vi "ReadCAlexFile.vi"(7 "ExtraWeight(kg)":cluster{"Thigh":dbl, "Shank":dbl}, 8 "error in (no error)":errorcluster, 10 "ExpData File Path":path, 11 "CAlexData2":refnum<class "CAlex2_Data.lvclass">) -> (0 "error out":errorcluster, 3 "CAlexData 2":refnum<class "CAlex2_Data.lvclass">, 5 "CAlexVersion":T1)   [LabVIEW 2016, in "CAlex2_Data.lvclass"]
uses:
  CAlex2_Data.lvclass
  E:/LabVIEW.git/CAlex2-controller-master/Sim&Process/DataProcess/ExpData/ExpData.lvclass
  Classes/CAlex2/TypeDef/CAlexVersion.ctl
  Classes/CAlex2/CAlex2.lvclass
  Classes/CAlex2/TypeDef/LowerBodyDim.ctl
  CAlex2_Data.lvclass/CAlex2_Data.ctl
  ExpData/ExpData.lvclass
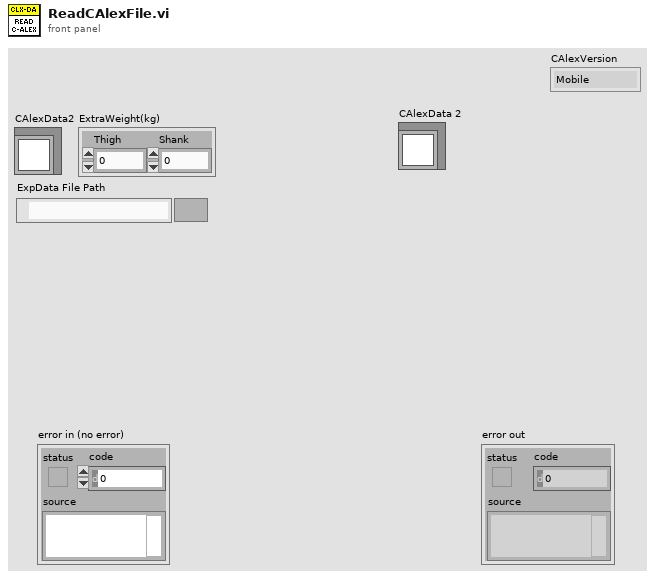
[diagram p1: front panel]
types:
  T1 = typedef "CAlex2.lvclass/CAlexVersion.ctl" = enum16{"Mobile", "Treadmill"}
  T2 = typedef "CAlex2.lvclass/LowerBodyDim.ctl" = cluster{"BodyDim":cluster{"ThighLt (m)":dbl, "ShankLt (m)":dbl, "HipWd (m)":dbl}, "BodyWt":cluster{"Thigh (kg)":dbl, "Shank (kg)":dbl}, "Cuff Loc":cluster{"HipCuffWd (m)":dbl, "HipCuffHt (m)":dbl, "HipFwdShift (m)":dbl, "ThighToKnee (m)":dbl, "ThighCuffDist (m)":dbl, "ShankToKnee (m)":dbl}}
  T3 = cluster{"[0]":dbl, "[1]":dbl, "[2]":dbl, "[3]":dbl, "[4]":dbl, "[5]":dbl}
  T4 = cluster{"array type (2D Dbl)[0]":dbl, "array type (2D Dbl)[1]":dbl, "array type (2D Dbl)[2]":dbl, "array type (2D Dbl)[3]":dbl, "array type (2D Dbl)[4]":dbl, "array type (2D Dbl)[5]":dbl}
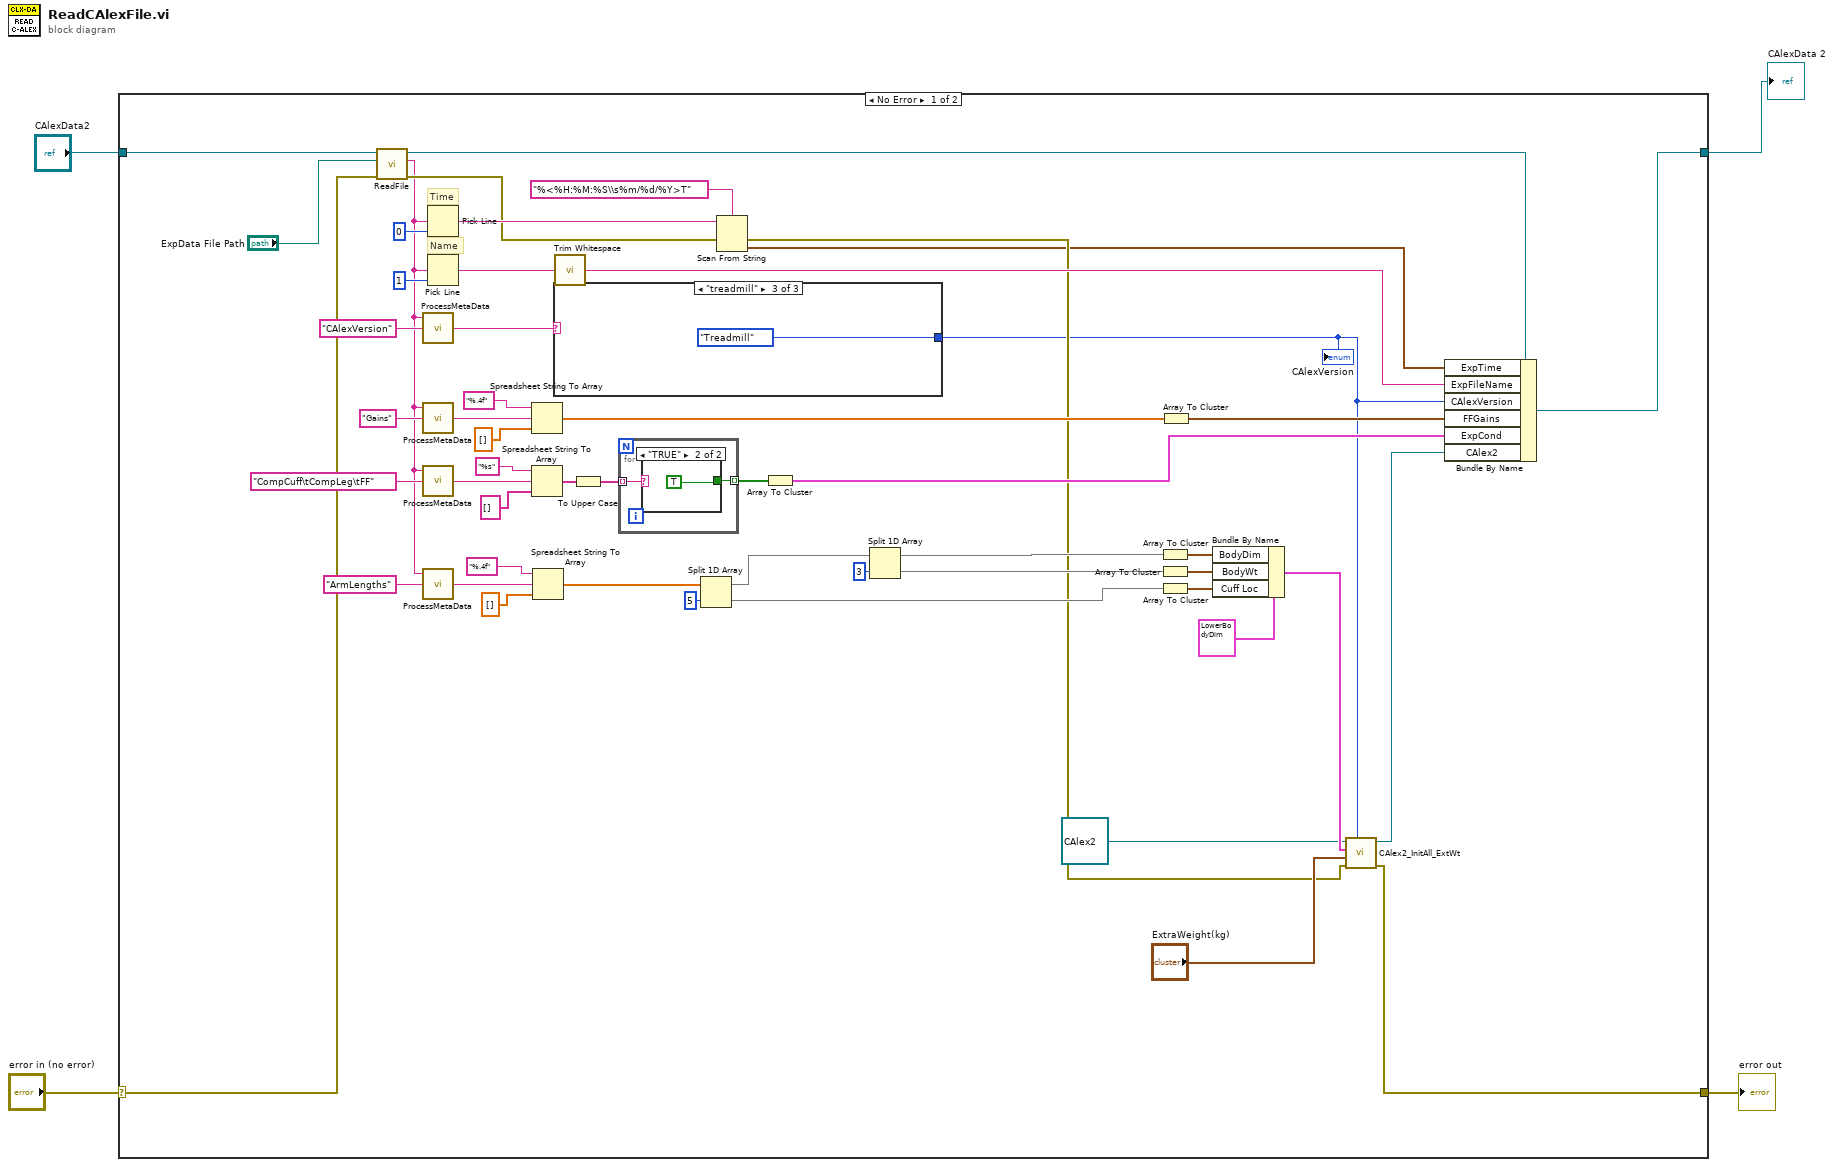
[diagram p0: block diagram]
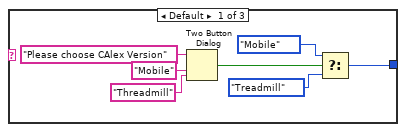
[diagram p2: hidden frame]
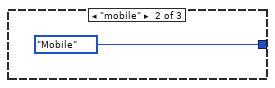
[diagram p3: hidden frame]
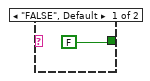
[diagram p4: hidden frame]
diagram:
  n1 = case shown="No Error" "error in (no error)" {
    selector: "error in (no error)" -> [w44 w71]
    tunnel: [w26 w71] -> w3
    tunnel: [w23 w70] -> w1
    tunnel: "CAlexData2" -> [w25 w70]
    frame No Error {
      # "Name"
      # "Time"
      n2 = call "ReadFile.vi"("error in (no error)"=w44, "ExpData File Path"="ExpData File Path", "ExpData In"=w25) -> ("error out"=w45:errorcluster, "MetaData"=w10:string, "ExpData Out"=w24:refnum<class "CAlex2_Data.lvclass">)  [unwired: 5 in, 1 out]
      n3 = call "ProcessMetaData.vi"("Header"="CAlexVersion", "MetaData"=w10) -> ("Data"=w6:string)  [unwired: 1 in]
      n4 = call "ProcessMetaData.vi"("Header"="Gains", "MetaData"=w10) -> ("Data"=w15:string)  [unwired: 1 in]
      n5 = call "ProcessMetaData.vi"("Header"="CompCuff\tCompLeg\tFF", "MetaData"=w10) -> ("Data"=w13:string)  [unwired: 1 in]
      n6 = call "ProcessMetaData.vi"("Header"="ArmLengths", "MetaData"=w10) -> ("Data"=w16:string)  [unwired: 1 in]
      n7 = Pick Line(multi-line string=w10, line index=0) -> (output string=w52:string)  [unwired: 1 in]
      n8 = Pick Line(multi-line string=w10, line index=1) -> (output string=w53:string)  [unwired: 1 in]
      n9 = Spreadsheet String To Array(format string="%.4f" ("format (%.3f)"), spreadsheet string=w15, array type (2D Dbl)=dbl[] []) -> (array=w43:dbl[])  [unwired: 1 in]
      n10 = Spreadsheet String To Array(format string="%s", spreadsheet string=w13, array type (2D Dbl)=string[] []) -> (array=w19:string[])  [unwired: 1 in]
      n11 = Spreadsheet String To Array(format string="%.4f" ("format (%.3f)"), spreadsheet string=w16, array type (2D Dbl)=dbl[] []) -> (array=w48:dbl[])  [unwired: 1 in]
      n12 = case shown="\"treadmill\"" w6 {
        tunnel: [w57 CAlexVersion."Mobile" ("CAlexVersion") CAlexVersion."Treadmill" ("CAlexVersion")] -> w5
        frame Default {
          n13 = Two Button Dialog(message="Please choose CAlex Version", 1:"Threadmill" ("F button name (\"Cancel\")"), 2:"Mobile" ("T button name (\"OK\")")) -> (T button?=w60:bool)
          n14 = Select(t=CAlexVersion."Mobile" ("CAlexVersion"), s=w60, f=CAlexVersion."Treadmill" ("CAlexVersion")) -> (s? t:f=w57:T1)
        }
        frame "mobile" {
        }
        frame "treadmill" {
        }
      }
      "CAlexVersion" <- w5
      n15 = call <vilib>:"Trim Whitespace.vi"("string"=w53) -> ("trimmed string"=w50:string)  [unwired: 1 in]
      n16 = To Upper Case(1:w19) -> (0:w18:string[])
      n17 = for {
        tunnel: w18 -> [w67] mode=indexing
        tunnel: [w66] -> w35 mode=indexing
        n18 = case shown="\"TRUE\"" w67 {
          tunnel: [FALSE TRUE] -> w66
          frame "FALSE", Default {
          }
          frame "TRUE" {
          }
        }
      }
      n19 = Split 1D Array(array=w48, index=5) -> (first subarray=w41:dbl[], second subarray=w38:dbl[])
      n20 = Scan From String(format string="%<%H:%M:%S\\s%m/%d/%Y>T", input string=w52, error in=w45) -> (error out=w27:errorcluster, output 1=w20:timestamp)  [unwired: 2 in, 2 out]
      n21 = Array To Cluster(array=w35) -> (cluster=w34:cluster{"[0]":bool, "[1]":bool, "[2]":bool})
      n22 = Split 1D Array(array=w41, index=3) -> (first subarray=w40:dbl[], second subarray=w39:dbl[])
      n23 = Array To Cluster(array=w40) -> (cluster=w33:cluster{"[0]":dbl, "[1]":dbl, "[2]":dbl})
      n24 = Array To Cluster(array=w39) -> (cluster=w32:cluster{"[0]":dbl, "[1]":dbl})
      n25 = Array To Cluster(array=w38) -> (cluster=w31:T3)
      n26 = Array To Cluster(array=w43) -> (cluster=w9:T4)
      n27 = Bundle By Name(cluster=T2 {"BodyDim"={"ThighLt (m)"=0.0, "ShankLt (m)"=0.0, "HipWd (m)"=0.0}, "BodyWt"={"Thigh (kg)"=0.0, "Shank (kg)"=0.0}, "Cuff Loc"={"HipCuffWd (m)"=0.0, "HipCuffHt (m)"=0.0, "HipFwdShift (m)"=0.0, "ThighToKnee (m)"=0.0, "ThighCuffDist (m)"=0.0, "ShankToKnee (m)"=0.0}} ("LegProperties"), "BodyDim"=w33, "BodyWt"=w32, "Cuff Loc"=w31) -> (w29:T2)
      n28 = call "CAlex2_InitAll_ExtWt.vi"("CAlexVersion"=w5, "error in (no error)"=w27, "ExtraWeight(kg)"="ExtraWeight(kg)", "LegProperties"=w29, "CAlex2 in"=refnum<class "CAlex2.lvclass"> refnum ("CAlex2")) -> ("error out"=w26:errorcluster, "CAlex2 out"=w30:refnum<class "CAlex2.lvclass">)  [unwired: 5 in]
      n29 = Bundle By Name(cluster=w24, "ExpTime"=w20, "ExpFileName"=w50, "CAlexVersion"=w5, "FFGains"=w9, "ExpCond"=w34, "CAlex2"=w30) -> (w23:refnum<class "CAlex2_Data.lvclass">)
    }
    frame Error {
    }
  }
  "error out" <- w3
  "CAlexData 2" <- w1
